vi "ReadWaveformAndMap.vi"(6 "length":i32, 8 "error in (no error)":errorcluster, 9 "index":i32, 10 "buffer location":u32, 11 "data group":string) -> (0 "error out":errorcluster, 1 "DVR element":T1, 2 "map":T2, 3 "waveforms":waveform(sgl)[](array[waveform]), 5 "found":bool)   [LabVIEW 2017, in "DVRBuffer.lvlib"]
uses:
  <vilib>/addons/InsightCM/Devices/Shared/Common/DVRBuffer/DVRBuffer.lvlib
  <vilib>/addons/PointValueMap/controls/PointMap.ctl
  <vilib>/addons/InsightCM/Devices/Shared/Common/DVRBuffer/controls/DVRElement.ctl
  <vilib>/addons/InsightCM/Devices/Shared/Common/DVRBuffer/controls/InternalDataType_waveformmap.ctl
  <vilib>/addons/PointValueMap/PointValueMap.lvlib
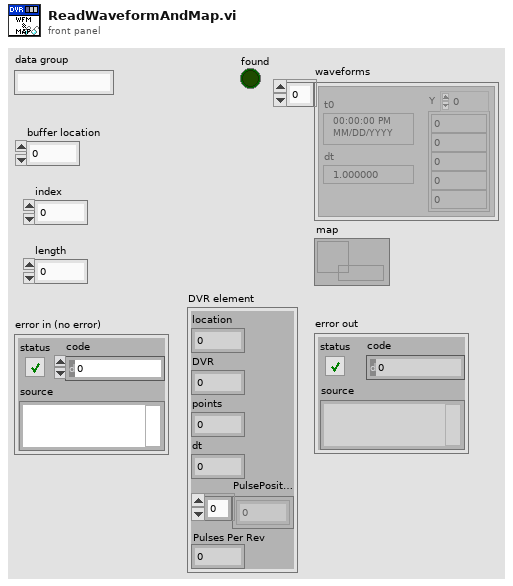
[diagram p1: front panel]
types:
  T1 = typedef "DVRBuffer.lvlib/DVRElement.ctl" = cluster{"location":u32, "DVR":u32, "points":i32, "dt":dbl, "PulsePositions":dbl[], "Pulses Per Rev":dbl}
  T2 = typedef "PointValueMap.lvlib/PointMap.ctl" = refnum<data-value>
  T3 = typedef "DVRBuffer.lvlib/InternalDataType_waveformmap.ctl" = cluster{"waveforms":waveform(sgl)[], "map":T2}
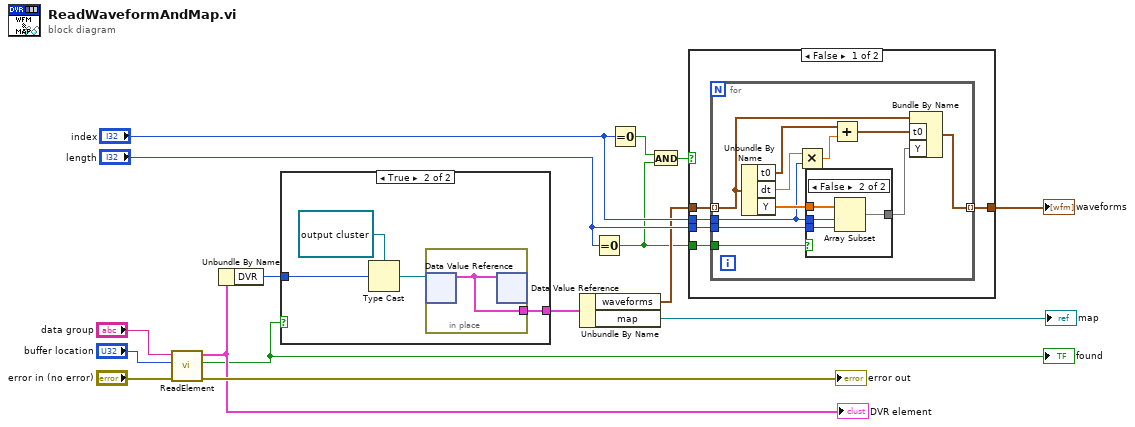
[diagram p0: block diagram]
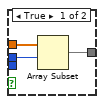
[diagram p2: hidden frame]
diagram:
  n1 = call <vilib>:"ReadElement.vi"("error in (no error)"="error in (no error)", "buffer location"="buffer location", "name"="data group") -> ("error out"=→"error out":errorcluster, "found"=w8:bool, "DVR element"=w10:T1)  [unwired: 6 in]
  "found" <- w8
  "DVR element" <- w10
  n2 = Unbundle By Name(w10) -> ("DVR"=w9:u32)
  n3 = case shown="True" w8 {
    tunnel: w9 -> [_ w20]
    tunnel: [_ w18] -> w12
    frame False {
    }
    frame True {
      n4 = Type Cast(type=refnum<data-value> refnum ("data value reference"), x=w20) -> (*(type *) &x=w19:refnum<data-value>)
      n5 = in-place {
        in-place-border: [w21] -> w18
        n6 = in-place-dvr #1(w19) -> (w21:T3)  [unwired: 1 out]
        n7 = in-place-dvr #1(w21) -> ()  [unwired: 2 out]
      }
    }
  }
  n8 = Unbundle By Name(w12) -> ("waveforms"=w5:waveform(sgl)[], "map"=→"map":T2)
  n9 = Equal To 0?(x="length") -> (x = 0?=w3:bool)
  n10 = Equal To 0?(x="index") -> (x = 0?=w2:bool)
  n11 = And(x=w2, y=w3) -> (x .and. y?=w1:bool)
  n12 = case shown="False" w1 {
    tunnel: w5 -> [w26 w45]
    tunnel: [w25 w45] -> w4
    tunnel: "length" -> [w24 _]
    tunnel: "index" -> [w23 _]
    tunnel: w3 -> [w22 _]
    frame False {
      n13 = for {
        tunnel: w26 -> [w34] mode=indexing
        tunnel: [w37] -> w25 mode=indexing
        tunnel: w23 -> [w30]
        tunnel: w22 -> [w33]
        tunnel: w24 -> [w32]
        n14 = Unbundle By Name(w34) -> ("t0"=w29:timestamp, "dt"=w31:dbl, "Y"=w36:sgl[])
        n15 = Multiply(x=w31, y=w30) -> (x*y=w28:dbl)
        n16 = case shown="False" w33 {
          tunnel: w36 -> [w40 w44]
          tunnel: [w39 w43] -> w35
          tunnel: w30 -> [w38 w42]
          tunnel: w32 -> [_ w41]
          frame True {
            n17 = Array Subset(array=w40, index=w38) -> (w39:sgl[])  [unwired: 1 in]
          }
          frame False {
            n18 = Array Subset(array=w44, index=w42, length=w41) -> (w43:sgl[])
          }
        }
        n19 = Add(x=w29, y=w28) -> (x+y=w27:timestamp)
        n20 = Bundle By Name(cluster=w34, "t0"=w27, "Y"=w35) -> (w37:waveform(sgl))
      }
    }
    frame True {
    }
  }
  "waveforms" <- w4
